vi "Periodic Tasks.vi"(8 "error in":errorcluster) -> ()   [LabVIEW 2015]
doc: "This VI runs in parallel to other tasks. It can contain as many user-defined periodic loops as you need. These can carry out PID or other sorts of timed response."
uses:
  PickupState.ctl
  ShootState.ctl
  TargetState.ctl
  <vilib>/Rock Robotics/WPI/Relay/WPI_RelayValue.ctl
  Robot Global Data.vi
  <vilib>/Rock Robotics/Network Tables/NT Write Numeric Array.vi
  <vilib>/Rock Robotics/WPI/Utilities/WPI_GetSetVariantRefNum.vi
  <vilib>/Rock Robotics/Network Tables/NT Read Numeric Array.vi
  <vilib>/Rock Robotics/WPI/RobotDrive/WPI_RobotDriveArcadeDrive_Standard(NoSaturation).vi
  <vilib>/Rock Robotics/Network Tables/NT Write Boolean Array.vi
  <vilib>/Rock Robotics/Network Tables/NT Read Number.vi
  <vilib>/Rock Robotics/Network Tables/NT Write Number.vi
panel:
  out "aligncount":dbl
  out "Distance (ft)":dbl
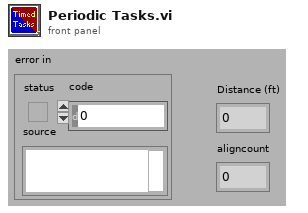
[diagram p1: front panel]
types:
  T1 = typedef "TargetState.ctl" = enum16{"Idle", "CheckVision", "AlignWithTarget", "MoveToTarget", "Wait", "ReAlign", "Stop", "Shoot", "Reset"}
  T2 = typedef "ShootState.ctl" = enum16{"Idle", "Startup", "Fire", "Shutdown", "Startup2"}
  T3 = typedef "PickupState.ctl" = enum16{"Idle", "Intake", "Continue", "Park", "Stop"}
  T4 = typedef "WPI_RelayDevRef.ctl" = cluster{"DevStatus":errorcluster, "Relay Channel":T5, "Relay Direction":T6}
  T5 = typedef "FPGA_DIORelayChannel.ctl" = enum8{"Relay 0", "Relay 1", "Relay 2", "Relay 3", "Invalid"}
  T6 = typedef "WPI_RelayDirection.ctl" = enum16{"Both directions", "Forward only", "Reverse only"}
  T7 = typedef "WPI_EncoderDevRef.ctl" = cluster{"DevStatus":errorcluster, "EncoderIndex":T8, "CounterIndex":T9, "DistancePerCount":dbl, "Decoding Type":T10}
  T8 = typedef "FPGA_EncoderIdx.ctl" = enum8{"Enc 0", "Enc 1", "Enc 2", "Enc 3", "Enc 4", "Enc 5", "Enc 6", "Enc 7", "Invalid"}
  T9 = typedef "FPGA_CounterCtrSystemIndex.ctl" = enum8{"Ctr 0", "Ctr 1", "Ctr 2", "Ctr 3", "Ctr 4", "Ctr 5", "Ctr 6", "Ctr 7", "Invalid"}
  T10 = typedef "WPI_EncoderType.ctl" = enum16{"1x", "2x", "4x"}
  T11 = typedef "WPI_GyroDevRef.ctl" = cluster{"DevStatus":errorcluster, "Analog Channel":T12, "Offset":dbl, "Gain (VoltsPerDegree/Second)":dbl, "Gyro Type":enum16{"Analog", "XRS450"}, "Handle":i32, "SPI Bus":T13, "Device Found":bool, "Sample Rate":dbl, "Calibrate On Open":bool}
  T12 = typedef "FPGA_AIChannel.ctl" = enum8{"AI 0", "AI 1", "AI 2", "AI 3", "AI MXP 0", "AI MXP 1", "AI MXP 2", "AI MXP 3", "Invalid"}
  T13 = typedef "spi_bus.ctl" = enum16{"SPI On-Board, CS0", "SPI On-Board, CS1", "SPI On-Board, CS2", "SPI On-Board, CS3", "SPI MXP", "Invalid"}
  T14 = typedef "WPI_DigitalInputDevRef.ctl" = cluster{"DevStatus":errorcluster, "DIO Channel":T15}
  T15 = typedef "FPGA_DIOChannel.ctl" = enum8{"DIO 0", "DIO 1", "DIO 2", "DIO 3", "DIO 4", "DIO 5", "DIO 6", "DIO 7", "DIO 8", "DIO 9", "DIO MXP 0", "DIO MXP 1", "DIO MXP 2", "DIO MXP 3", "DIO MXP 4", "DIO MXP 5", "DIO MXP 6", "DIO MXP 7", "DIO MXP 8", "DIO MXP 9", "DIO MXP 10", "DIO MXP 11", "DIO MXP 12", "DIO MXP 13", "DIO MXP 14", "DIO MXP 15", "Invalid"}
  T16 = typedef "WPI_RobotDriveDevRef.ctl" = cluster{"DevStatus":errorcluster, "Motors[]":T17[], "Square Inputs":bool, "Max Output":dbl}
  T17 = typedef "WPI_MotorControlDeviceRef.ctl" = cluster{"DeviceStatus":errorcluster, "Type":T18, "PWM":cluster{"PWM Channel":T19, "DeadBand":T20}, "CAN":cluster{"Device Number":u8, "Control Mode":T21, "Semaphore":T22, "Max Vout":dbl, "TalonSRX Control Mode":T23}, "Invert":bool}
  T18 = typedef "WPI_MotorControlType.ctl" = enum16{"PWM", "CAN", "CANTalonSRX"}
  T19 = typedef "FPGA_DIOPWMChannel.ctl" = enum8{"PWM 0", "PWM 1", "PWM 2", "PWM 3", "PWM 4", "PWM 5", "PWM 6", "PWM 7", "PWM 8", "PWM 9", "PWM MXP 0", "PWM MXP 1", "PWM MXP 2", "PWM MXP 3", "PWM MXP 4", "PWM MXP 5", "PWM MXP 6", "PWM MXP 7", "PWM MXP 8", "PWM MXP 9", "Invalid"}
  T20 = typedef "WPI_PWMDeadband.ctl" = cluster{"Name":string, "maxPositivePwm":i32, "minPositivePwm":i32, "centerPwm":i32, "maxNegativePwm":i32, "minNegativePwm":i32, "angularRange":u16}
  T21 = typedef "WPI_CANJaguar_ControlMode.ctl" = enum8{"Percent VBus", "Current", "Speed", "Position", "Voltage"}
  T22 = typedef "Semaphore RefNum" = refnum<k1>
  T23 = typedef "WPI_CANTalonSRX_APIControlMode.ctl" = enum8{"Percent VBus", "Speed", "Position", "Slave", "Unchanged / Invalid", "Voltage Compensation", "Current", "Motion Profile"}
  T24 = typedef "WPI_RelayValue.ctl" = enum16{"Off", "On", "Forward", "Reverse"}
  T25 = cluster{"Distance (ft)":dbl, "Center":cluster{dbl, dbl}, "Normalized Rect":cluster{"Numeric":dbl, "Numeric 2":dbl, "Numeric 3":dbl, "Numeric 5":dbl}}[]
  T26 = cluster{"Distance (ft)":dbl, "Center":cluster{dbl, dbl}, "Normalized Rect":cluster{"Numeric":dbl, "Numeric 2":dbl, "Numeric 3":dbl, "Numeric 5":dbl}}
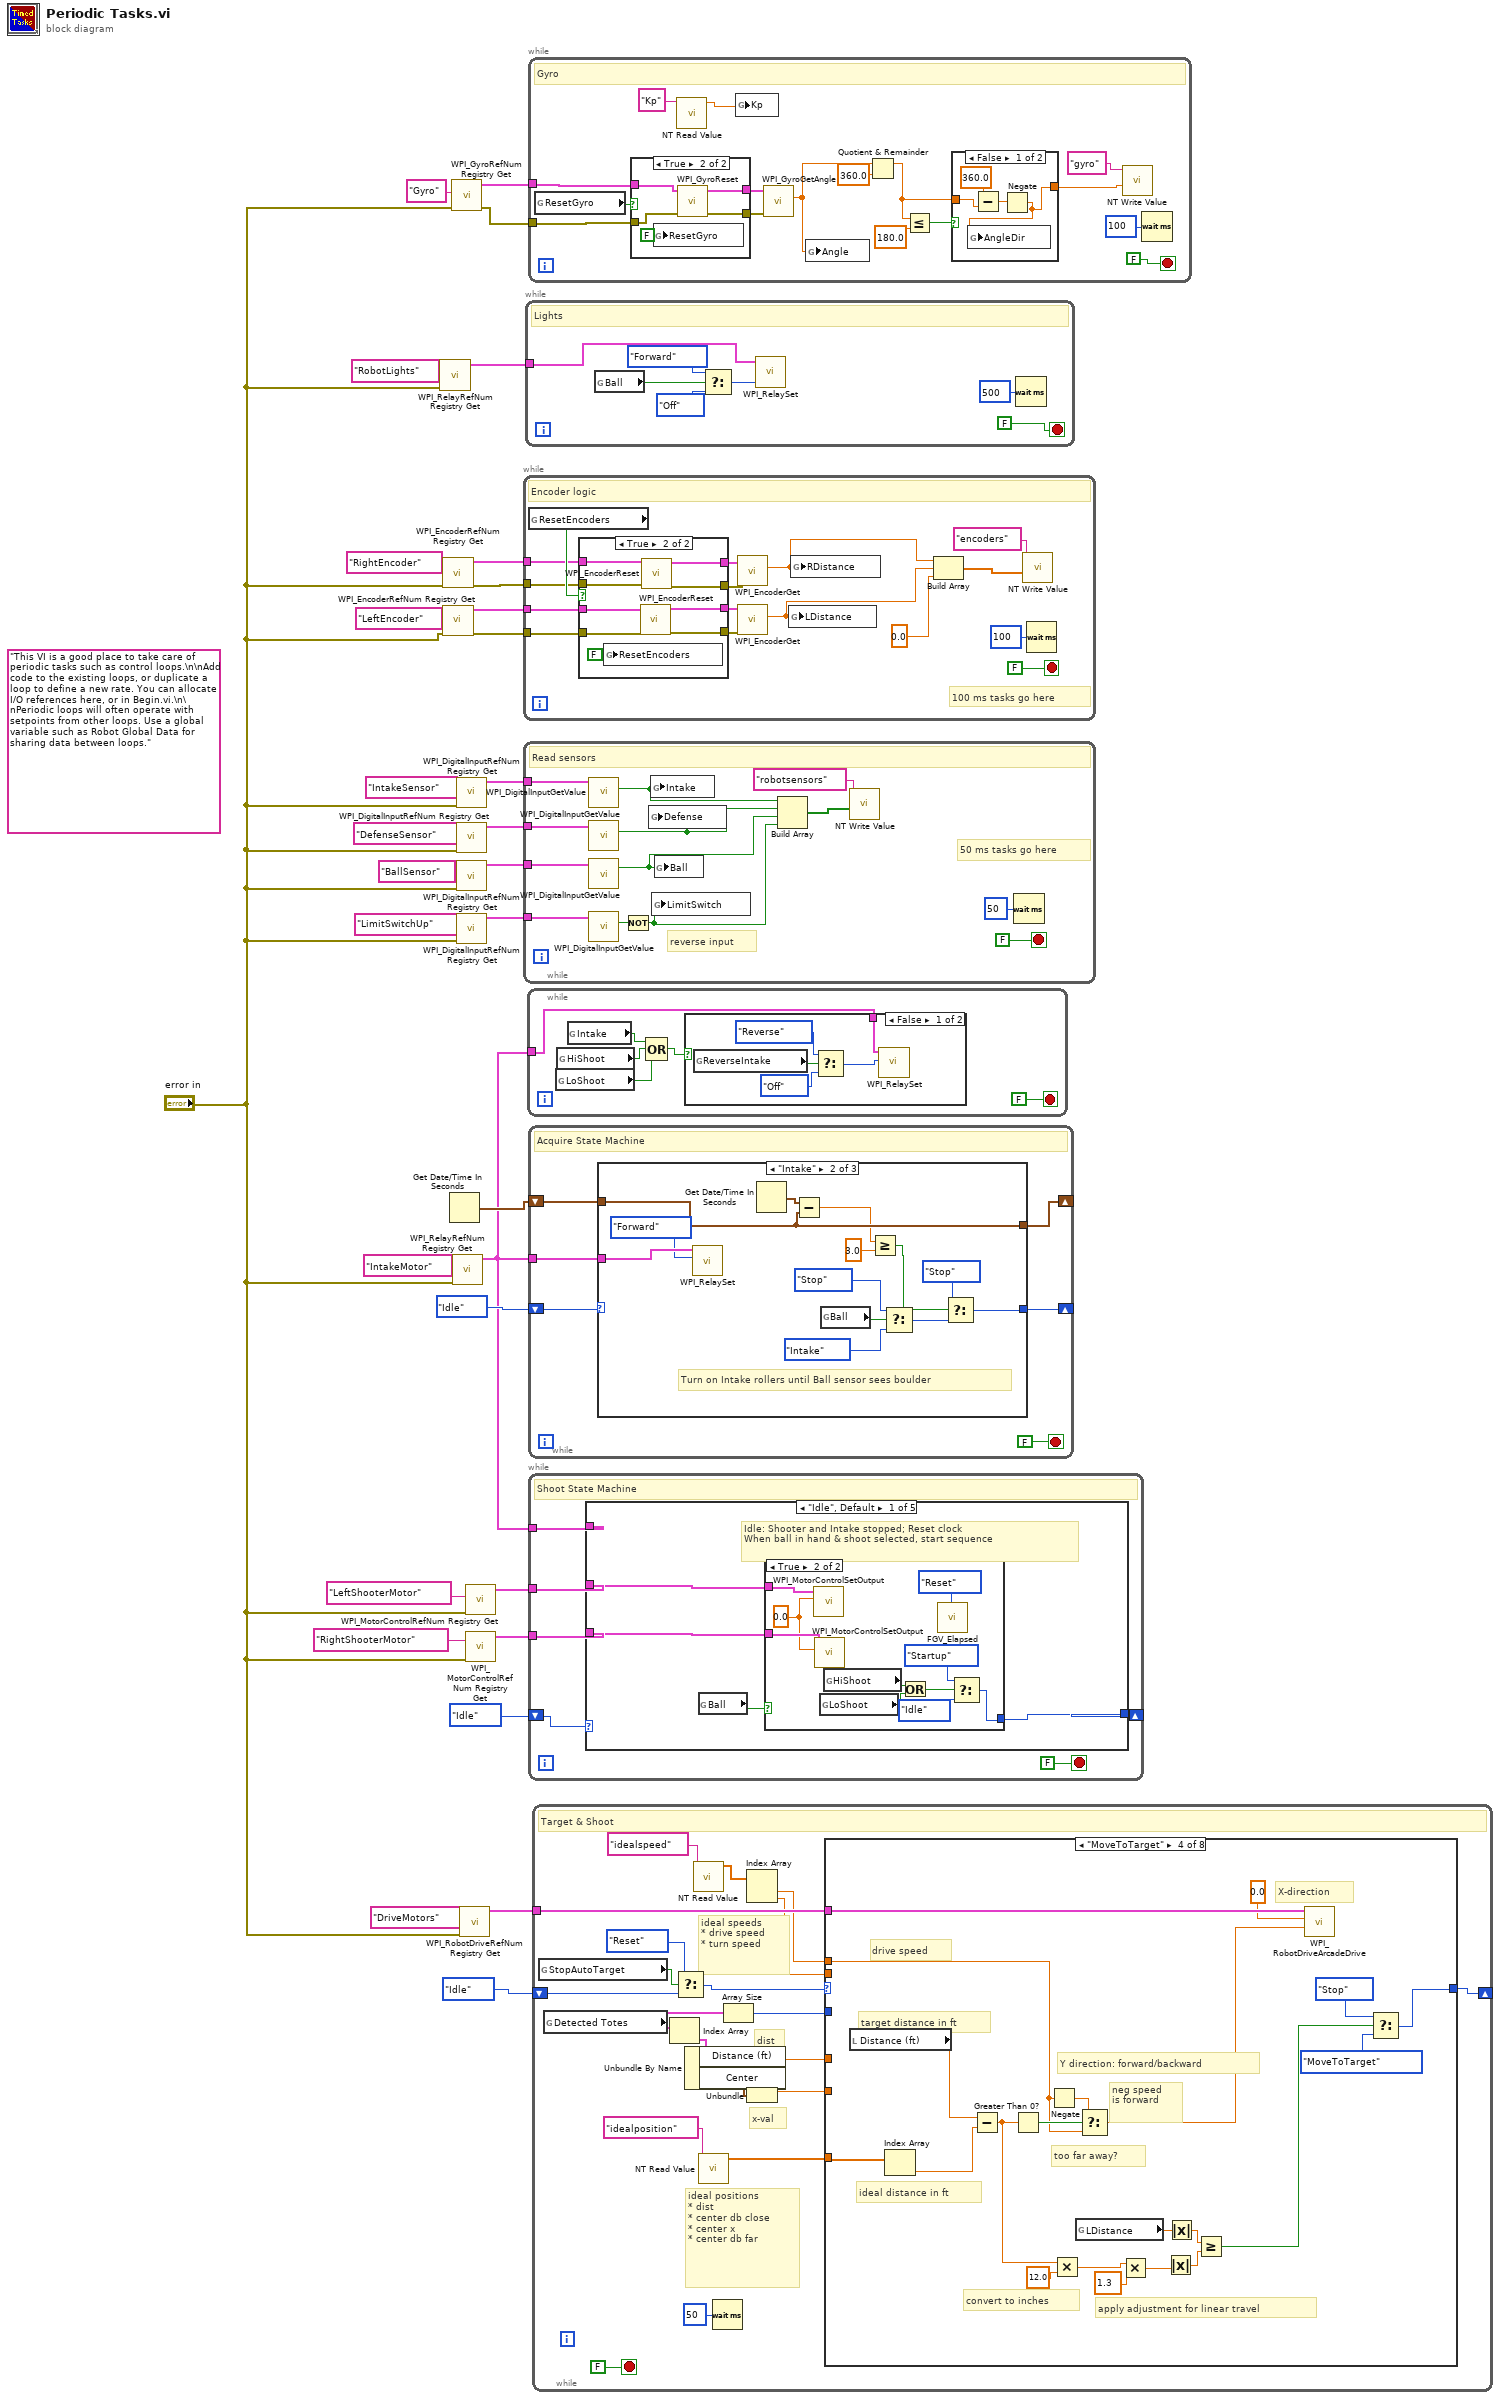
[diagram p0: block diagram]
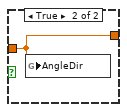
[diagram p2: hidden frame]
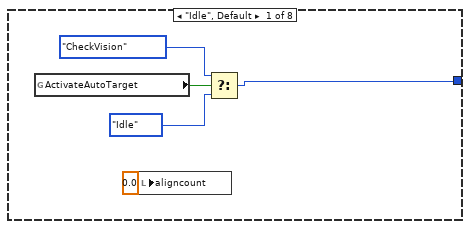
[diagram p5: hidden frame]
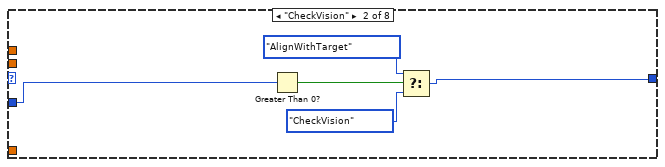
[diagram p6: hidden frame]
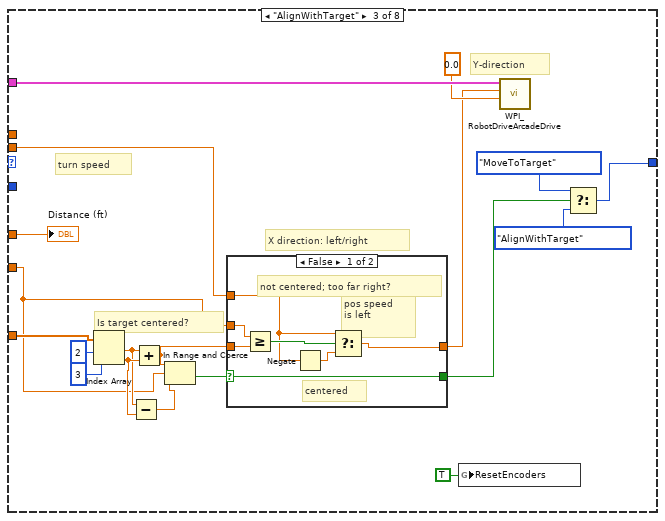
[diagram p7: hidden frame]
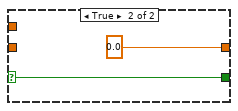
[diagram p8: hidden frame]
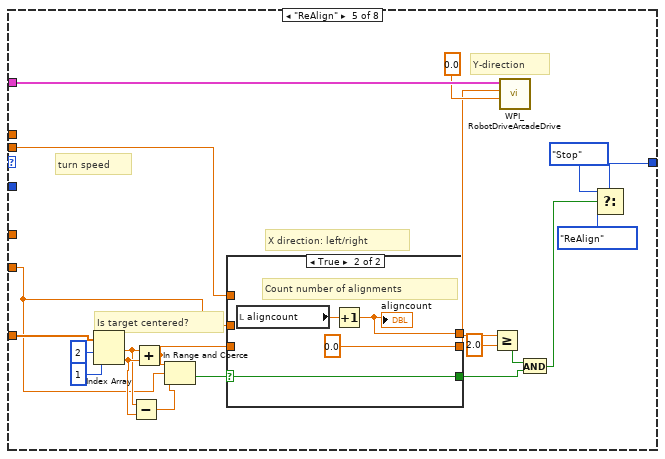
[diagram p9: hidden frame]
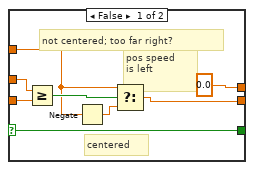
[diagram p10: hidden frame]
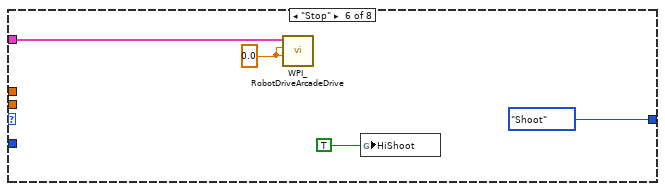
[diagram p11: hidden frame]
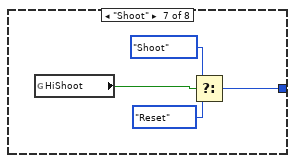
[diagram p12: hidden frame]
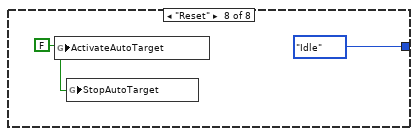
[diagram p13: hidden frame]
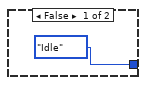
[diagram p14: hidden frame]
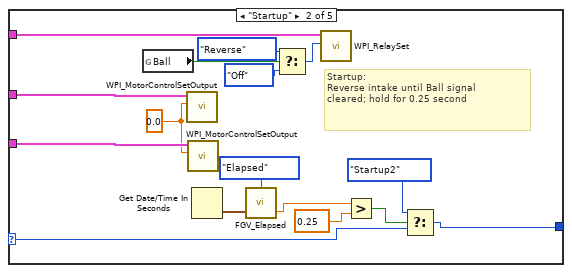
[diagram p15: hidden frame]
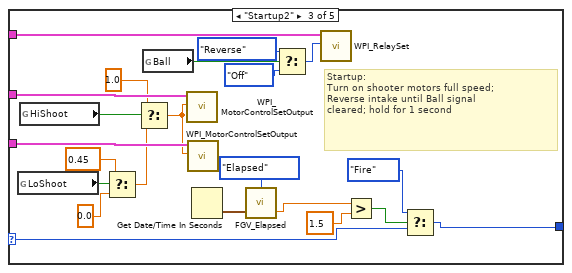
[diagram p16: hidden frame]
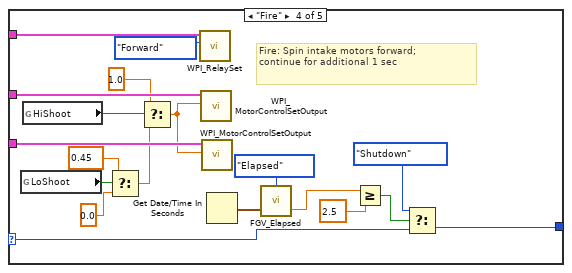
[diagram p17: hidden frame]
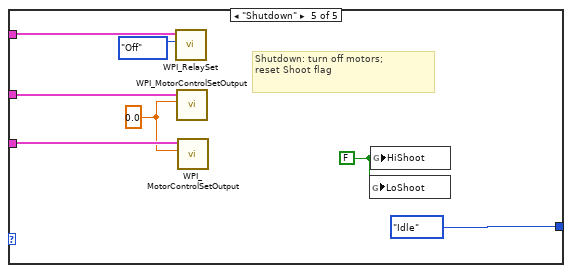
[diagram p18: hidden frame]
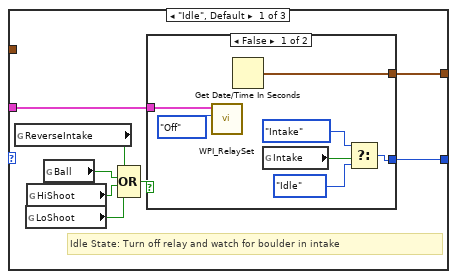
[diagram p19: hidden frame]
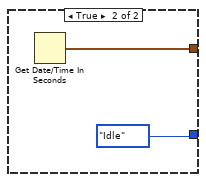
[diagram p20: hidden frame]
diagram:
  (unwired) "This VI is a good place to take care of periodic tasks such as control loops.\n\nAdd code to the existing loops, or duplicate a loop to define a new rate. You can allocate I/O references here, or in Begin.vi.\n\nPeriodic loops will often operate with setpoints from other loops. Use a global variable such as Robot Global Data for sharing data between loops."
  n1 = call <vilib>:"WPI_RelayRefNum Registry Get.vi"("error in (no error)"="error in", "refnum name"="RobotLights") -> ("RelayDevRef"=w14:T4)  [unwired: 8 in, 1 out]
  n2 = call <vilib>:"WPI_EncoderRefNum Registry Get.vi"("error in (no error)"="error in", "refnum name"="RightEncoder") -> ("error out"=w30:errorcluster, "EncoderDevRef"=w31:T7)  [unwired: 8 in]
  n3 = call <vilib>:"WPI_EncoderRefNum Registry Get.vi"("error in (no error)"="error in", "refnum name"="LeftEncoder") -> ("error out"=w29:errorcluster, "EncoderDevRef"=w32:T7)  [unwired: 8 in]
  n4 = Get Date/Time In Seconds() -> (seconds since 1Jan1904=w6:timestamp)
  n5 = call <vilib>:"WPI_GyroRefNum Registry Get.vi"("error in (no error)"="error in", "refnum name"="Gyro") -> ("error out"=w2:errorcluster, "GyroDevRef"=w3:T11)  [unwired: 8 in]
  n6 = call <vilib>:"WPI_RelayRefNum Registry Get.vi"("error in (no error)"="error in", "refnum name"="IntakeMotor") -> ("RelayDevRef"=w5:T4)  [unwired: 8 in, 1 out]
  n7 = call <vilib>:"WPI_DigitalInputRefNum Registry Get.vi"("error in (no error)"="error in", "refnum name"="IntakeSensor") -> ("DigitalInputDevRef"=w24:T14)  [unwired: 8 in, 1 out]
  n8 = call <vilib>:"WPI_DigitalInputRefNum Registry Get.vi"("error in (no error)"="error in", "refnum name"="DefenseSensor") -> ("DigitalInputDevRef"=w10:T14)  [unwired: 8 in, 1 out]
  n9 = call <vilib>:"WPI_DigitalInputRefNum Registry Get.vi"("error in (no error)"="error in", "refnum name"="BallSensor") -> ("DigitalInputDevRef"=w16:T14)  [unwired: 8 in, 1 out]
  n10 = call <vilib>:"WPI_DigitalInputRefNum Registry Get.vi"("error in (no error)"="error in", "refnum name"="LimitSwitchUp") -> ("DigitalInputDevRef"=w7:T14)  [unwired: 8 in, 1 out]
  n11 = call <vilib>:"WPI_RobotDriveRefNum Registry Get.vi"("error in (no error)"="error in", "refnum name"="DriveMotors") -> ("RobotDriveDevRef"=w11:T16)  [unwired: 8 in, 1 out]
  n12 = call <vilib>:"WPI_MotorControlRefNum Registry Get.vi"("error in (no error)"="error in", "refnum name"="LeftShooterMotor") -> ("MotorControlDevRef"=w19:T17)  [unwired: 8 in, 1 out]
  n13 = call <vilib>:"WPI_MotorControlRefNum Registry Get.vi"("error in (no error)"="error in", "refnum name"="RightShooterMotor") -> ("MotorControlDevRef"=w18:T17)  [unwired: 8 in, 1 out]
  n14 = while {
    tunnel: w32 -> [w37]
    tunnel: w31 -> [w41]
    tunnel: w30 -> [w39]
    tunnel: w29 -> [w36]
    stop <- FALSE stop-if-true
    # "100 ms tasks go here"
    # "Encoder logic"
    n15 = global read "Robot Global Data.vi" "ResetEncoders"() -> (w42:bool)
    n16 = case shown="True" w42 {
      tunnel: w41 -> [w52 w61]
      tunnel: [w52 w60] -> w40
      tunnel: w39 -> [w51 w59]
      tunnel: [w51 w58] -> w38
      tunnel: w37 -> [w50 w57]
      tunnel: w36 -> [w49 w56]
      tunnel: [w50 w55] -> w35
      tunnel: [w49 w54] -> w34
      frame False {
      }
      frame True {
        n17 = global write "Robot Global Data.vi" "ResetEncoders"(FALSE) -> ()
        n18 = call <vilib>:"WPI_EncoderReset.vi"("error in (no error)"=w56, "EncoderDevRef"=w57) -> ("error out"=w54:errorcluster, "EncoderDevRef"=w55:T7)  [unwired: 8 in]
        n19 = call <vilib>:"WPI_EncoderReset.vi"("error in (no error)"=w59, "EncoderDevRef"=w61) -> ("error out"=w58:errorcluster, "EncoderDevRef"=w60:T7)  [unwired: 8 in]
      }
    }
    n20 = call <vilib>:"WPI_EncoderGet.vi"("error in (no error)"=w38, "EncoderDevRef"=w40) -> ("Distance"=w44:dbl)  [unwired: 4 in, 5 out]
    n21 = call <vilib>:"WPI_EncoderGet.vi"("error in (no error)"=w34, "EncoderDevRef"=w35) -> ("Distance"=w43:dbl)  [unwired: 4 in, 5 out]
    n22 = global write "Robot Global Data.vi" "LDistance"(w43) -> ()
    n23 = global write "Robot Global Data.vi" "RDistance"(w44) -> ()
    n24 = Build Array(w44, w43, 0.0) -> (w46:dbl[])
    n25 = call-poly <vilib>:"NT Write Value.vi"("Numeric Array"=w46, "Name"="encoders") -> ()  [unwired: 9 in, 1 out]
    n26 = Wait (ms)(milliseconds to wait=u32 100) -> ()  [unwired: 1 out]
  }
  n27 = while {
    tunnel: w24 -> [w72]
    tunnel: w16 -> [w68]
    tunnel: w10 -> [w66]
    tunnel: w7 -> [w65]
    stop <- FALSE stop-if-true
    # "reverse input"
    # "50 ms tasks go here"
    # "Read sensors"
    n28 = call <vilib>:"WPI_DigitalInputGetValue.vi"("DigitalInputDevRef"=w72) -> ("Value"=w71:bool)  [unwired: 8 in, 2 out]
    n29 = call <vilib>:"WPI_DigitalInputGetValue.vi"("DigitalInputDevRef"=w66) -> ("Value"=w63:bool)  [unwired: 8 in, 2 out]
    n30 = call <vilib>:"WPI_DigitalInputGetValue.vi"("DigitalInputDevRef"=w68) -> ("Value"=w67:bool)  [unwired: 8 in, 2 out]
    n31 = call <vilib>:"WPI_DigitalInputGetValue.vi"("DigitalInputDevRef"=w65) -> ("Value"=w64:bool)  [unwired: 8 in, 2 out]
    n32 = Not(x=w64) -> (.not. x?=w62:bool)
    n33 = global write "Robot Global Data.vi" "Defense"(w63) -> ()
    n34 = global write "Robot Global Data.vi" "Intake"(w71) -> ()
    n35 = global write "Robot Global Data.vi" "LimitSwitch"(w62) -> ()
    n36 = global write "Robot Global Data.vi" "Ball"(w67) -> ()
    n37 = Build Array(w71, w63, w67, w62) -> (w70:bool[])
    n38 = call-poly <vilib>:"NT Write Value.vi"("Boolean Array"=w70, "Name"="robotsensors") -> ()  [unwired: 9 in, 1 out]
    n39 = Wait (ms)(milliseconds to wait=u32 50) -> ()  [unwired: 1 out]
  }
  n40 = while {
    tunnel: w14 -> [w78]
    stop <- FALSE stop-if-true
    # "Lights"
    n41 = global read "Robot Global Data.vi" "Ball"() -> (w77:bool)
    n42 = Select(t=WPI_RelayValue."Forward" ("RelayValue"), s=w77, f=WPI_RelayValue."Off" ("RelayValue")) -> (s? t:f=w81:T24)
    n43 = call <vilib>:"WPI_RelaySet.vi"("RelayValue"=w81, "RelayDevRef"=w78) -> ()  [unwired: 8 in, 2 out]
    n44 = Wait (ms)(milliseconds to wait=u32 500) -> ()  [unwired: 1 out]
  }
  n45 = while {
    tunnel: w5 -> [w86]
    stop <- FALSE stop-if-true
    n46 = global read "Robot Global Data.vi" "LoShoot"() -> (w85:bool)
    n47 = global read "Robot Global Data.vi" "HiShoot"() -> (w84:bool)
    n48 = global read "Robot Global Data.vi" "Intake"() -> (w82:bool)
    n49 = Compound Arithmetic op=OR(w82, w84, w85) -> (w83:bool)
    n50 = case shown="False" w83 {
      tunnel: w86 -> [w92 _]
      frame False {
        n51 = global read "Robot Global Data.vi" "ReverseIntake"() -> (w88:bool)
        n52 = Select(t=WPI_RelayValue."Reverse" ("RelayValue"), s=w88, f=WPI_RelayValue."Off" ("RelayValue")) -> (s? t:f=w89:T24)
        n53 = call <vilib>:"WPI_RelaySet.vi"("RelayValue"=w89, "RelayDevRef"=w92) -> ()  [unwired: 8 in, 2 out]
      }
      frame True {
      }
    }
  }
  n54 = while {
    tunnel: w3 -> [w108]
    tunnel: w2 -> [w106]
    stop <- FALSE stop-if-true
    # "Gyro"
    n55 = global read "Robot Global Data.vi" "ResetGyro"() -> (w104:bool)
    n56 = case shown="True" w104 {
      tunnel: w108 -> [w114 w120]
      tunnel: [w114 w119] -> w107
      tunnel: w106 -> [w115 w118]
      tunnel: [w115 w117] -> w105
      frame False {
      }
      frame True {
        n57 = global write "Robot Global Data.vi" "ResetGyro"(FALSE) -> ()
        n58 = call <vilib>:"WPI_GyroReset.vi"("error in"=w118, "GyroDevRef"=w120) -> ("error out"=w117:errorcluster, "GyroDevRef"=w119:T11)  [unwired: 8 in]
      }
    }
    n59 = call-poly <vilib>:"NT Read Value.vi"("Name"="Kp") -> ("Numeric"=w93:dbl)  [unwired: 9 in, 1 out]
    n60 = global write "Robot Global Data.vi" "Kp"(w93) -> ()
    n61 = call <vilib>:"WPI_GyroGetAngle.vi"("error in"=w105, "GyroDevRef"=w107) -> ("Angle"=w101:dbl)  [unwired: 5 in, 4 out]
    n62 = global write "Robot Global Data.vi" "Angle"(w101) -> ()
    n63 = Quotient & Remainder(x=w101, y=360.0) -> (x-y*floor(x/y)=w96:dbl)  [unwired: 1 out]
    n64 = Less Or Equal?(x=w96, y=180.0) -> (x <= y?=w98:bool)
    n65 = case shown="False" w98 {
      tunnel: w96 -> [w111 w113]
      tunnel: [w109 w113] -> w95
      frame False {
        n66 = Subtract(x=360.0 ("y"), y=w111) -> (x-y=w110:dbl)
        n67 = Negate(x=w110) -> (-x=w109:dbl)
        n68 = global write "Robot Global Data.vi" "AngleDir"(w109) -> ()
      }
      frame True {
        n69 = global write "Robot Global Data.vi" "AngleDir"(w113) -> ()
      }
    }
    n70 = call-poly <vilib>:"NT Write Value.vi"("Numeric"=w95, "Name"="gyro") -> ()  [unwired: 9 in, 1 out]
    n71 = Wait (ms)(milliseconds to wait=u32 100) -> ()  [unwired: 1 out]
  }
  n72 = while {
    shift-right: [w123] -> _
    shift-left: PickupState."Idle" ("PickupState") -> [w125]
    tunnel: w5 -> [w124]
    shift-right: [w122] -> _
    shift-left: w6 -> [w121]
    stop <- FALSE stop-if-true
    # "Acquire State Machine"
    n73 = case shown="\"Intake\"" w125 {
      tunnel: w124 -> [w133 w156 w160]
      tunnel: [w134 w151 PickupState."Idle" ("PickupState")] -> w123
      tunnel: [w132 w147 w157] -> w122
      tunnel: w121 -> [_ w147 w157]
      frame "Idle", Default {
        # "Idle State: Turn off relay and watch for boulder in intake"
        n74 = global read "Robot Global Data.vi" "ReverseIntake"() -> (w127:bool)
        n75 = global read "Robot Global Data.vi" "LoShoot"() -> (w128:bool)
        n76 = global read "Robot Global Data.vi" "HiShoot"() -> (w129:bool)
        n77 = global read "Robot Global Data.vi" "Ball"() -> (w130:bool)
        n78 = Compound Arithmetic op=OR(w127, w130, w129, w128) -> (w131:bool)
        n79 = case shown="False" w131 {
          tunnel: [w140 PickupState."Idle" ("PickupState")] -> w134
          tunnel: w133 -> [w138 _]
          tunnel: [w135 w142] -> w132
          frame False {
            n80 = call <vilib>:"WPI_RelaySet.vi"("RelayValue"=WPI_RelayValue."Off", "RelayDevRef"=w138) -> ()  [unwired: 8 in, 2 out]
            n81 = Get Date/Time In Seconds() -> (seconds since 1Jan1904=w135:timestamp)
            n82 = global read "Robot Global Data.vi" "Intake"() -> (w141:bool)
            n83 = Select(t=PickupState."Intake" ("PickupState"), s=w141, f=PickupState."Idle" ("PickupState")) -> (s? t:f=w140:T3)
          }
          frame True {
            n84 = Get Date/Time In Seconds() -> (seconds since 1Jan1904=w142:timestamp)
          }
        }
      }
      frame "Intake" {
        # "Turn on Intake rollers until Ball sensor sees boulder"
        n85 = call <vilib>:"WPI_RelaySet.vi"("RelayValue"=WPI_RelayValue."Forward", "RelayDevRef"=w156) -> ()  [unwired: 8 in, 2 out]
        n86 = Get Date/Time In Seconds() -> (seconds since 1Jan1904=w148:timestamp)
        n87 = Subtract(x=w148, y=w147) -> (x-y=w146:dbl)
        n88 = global read "Robot Global Data.vi" "Ball"() -> (w154:bool)
        n89 = Greater Or Equal?(x=w146, y=3.0) -> (x >= y?=w144:bool)
        n90 = Select(t=PickupState."Stop" ("PickupState"), s=w154, f=PickupState."Intake" ("PickupState")) -> (s? t:f=w150:T3)
        n91 = Select(t=PickupState."Stop" ("PickupState"), s=w144, f=w150) -> (s? t:f=w151:T3)
      }
      frame "Stop" {
        # "Stop the motor"
        n92 = call <vilib>:"WPI_RelaySet.vi"("RelayValue"=WPI_RelayValue."Off", "RelayDevRef"=w160) -> ()  [unwired: 8 in, 2 out]
      }
    }
  }
  n93 = while {
    shift-right: [w162] -> _
    shift-left: ShootState."Idle" ("ShootState") -> [w166]
    tunnel: w5 -> [w161]
    tunnel: w19 -> [w164]
    tunnel: w18 -> [w163]
    stop <- FALSE stop-if-true
    # "Shoot State Machine"
    n94 = case shown="\"Idle\", Default" w166 {
      selector: w166 -> [_ w193 w215 w231 _]
      tunnel: w164 -> [w170 w197 w219 w238 w245]
      tunnel: w163 -> [w169 w196 w218 w237 w244]
      tunnel: [w168 w192 w214 w233 ShootState."Idle" ("ShootState")] -> w162
      tunnel: w161 -> [_ w187 w209 w236 w243]
      frame "Idle", Default {
        # "Idle: Shooter and Intake stopped; Reset clock\nWhen ball in hand & shoot selected, start sequence"
        n95 = global read "Robot Global Data.vi" "Ball"() -> (w167:bool)
        n96 = case shown="True" w167 {
          tunnel: w170 -> [_ w181]
          tunnel: w169 -> [_ w180]
          tunnel: [ShootState."Idle" ("ShootState") w178] -> w168
          frame False {
          }
          frame True {
            w179 = 0.0 ("Output")
            n97 = call <vilib>:"WPI_MotorControlSetOutput.vi"("Output"=w179, "MotorControlDevRef"=w181) -> ()  [unwired: 7 in, 3 out]
            n98 = call <vilib>:"WPI_MotorControlSetOutput.vi"("Output"=w179, "MotorControlDevRef"=w180) -> ()  [unwired: 7 in, 3 out]
            n99 = global read "Robot Global Data.vi" "LoShoot"() -> (w173:bool)
            n100 = global read "Robot Global Data.vi" "HiShoot"() -> (w174:bool)
            n101 = Or(x=w174, y=w173) -> (x .or. y?=w172:bool)
            n102 = call "FGV_Elapsed.vi"("Function"=enum16{"Elapsed", "Reset"}."Reset") -> ()  [unwired: 1 in, 1 out]
            n103 = Select(t=ShootState."Startup" ("ShootState"), s=w172, f=ShootState."Idle" ("ShootState")) -> (s? t:f=w178:T2)
          }
        }
      }
      frame "Startup" {
        w182 = 0.0 ("f")
        # "Startup:\nReverse intake until Ball signal\ncleared; hold for 0.25 second"
        n104 = global read "Robot Global Data.vi" "Ball"() -> (w186:bool)
        n105 = call <vilib>:"WPI_MotorControlSetOutput.vi"("Output"=w182, "MotorControlDevRef"=w197) -> ()  [unwired: 7 in, 3 out]
        n106 = call <vilib>:"WPI_MotorControlSetOutput.vi"("Output"=w182, "MotorControlDevRef"=w196) -> ()  [unwired: 7 in, 3 out]
        n107 = Get Date/Time In Seconds() -> (seconds since 1Jan1904=w190:timestamp)
        n108 = call "FGV_Elapsed.vi"("Function"=enum16{"Elapsed", "Reset"}."Elapsed", "DateTime"=w190) -> ("Elapsed"=w189:dbl)
        n109 = Select(t=WPI_RelayValue."Reverse" ("RelayValue"), s=w186, f=WPI_RelayValue."Off" ("RelayValue")) -> (s? t:f=w183:T24)
        n110 = call <vilib>:"WPI_RelaySet.vi"("RelayValue"=w183, "RelayDevRef"=w187) -> ()  [unwired: 8 in, 2 out]
        n111 = Greater?(x=w189, y=0.25) -> (0:w194:bool)
        n112 = Select(t=ShootState."Startup2" ("ShootState"), s=w194, f=w193) -> (s? t:f=w192:T2)
      }
      frame "Startup2" {
        # "Startup:\nTurn on shooter motors full speed;\nReverse intake until Ball signal\ncleared; hold for 1 second"
        n113 = global read "Robot Global Data.vi" "LoShoot"() -> (w202:bool)
        n114 = global read "Robot Global Data.vi" "HiShoot"() -> (w204:bool)
        n115 = Select(t=0.45, s=w202, f=0.0) -> (s? t:f=w200:dbl)
        n116 = Select(t=1.0, s=w204, f=w200) -> (s? t:f=w198:dbl)
        n117 = global read "Robot Global Data.vi" "Ball"() -> (w208:bool)
        n118 = call <vilib>:"WPI_MotorControlSetOutput.vi"("Output"=w198, "MotorControlDevRef"=w219) -> ()  [unwired: 7 in, 3 out]
        n119 = call <vilib>:"WPI_MotorControlSetOutput.vi"("Output"=w198, "MotorControlDevRef"=w218) -> ()  [unwired: 7 in, 3 out]
        n120 = Get Date/Time In Seconds() -> (seconds since 1Jan1904=w212:timestamp)
        n121 = call "FGV_Elapsed.vi"("Function"=enum16{"Elapsed", "Reset"}."Elapsed", "DateTime"=w212) -> ("Elapsed"=w211:dbl)
        n122 = Select(t=WPI_RelayValue."Reverse" ("RelayValue"), s=w208, f=WPI_RelayValue."Off" ("RelayValue")) -> (s? t:f=w205:T24)
        n123 = call <vilib>:"WPI_RelaySet.vi"("RelayValue"=w205, "RelayDevRef"=w209) -> ()  [unwired: 8 in, 2 out]
        n124 = Greater?(x=w211, y=1.5) -> (0:w216:bool)
        n125 = Select(t=ShootState."Fire" ("ShootState"), s=w216, f=w215) -> (s? t:f=w214:T2)
      }
      frame "Fire" {
        # "Fire: Spin intake motors forward;\ncontinue for additional 1 sec"
        n126 = global read "Robot Global Data.vi" "LoShoot"() -> (w224:bool)
        n127 = global read "Robot Global Data.vi" "HiShoot"() -> (w226:bool)
        n128 = Select(t=0.45, s=w224, f=0.0) -> (s? t:f=w222:dbl)
        n129 = Select(t=1.0, s=w226, f=w222) -> (s? t:f=w221:dbl)
        n130 = call <vilib>:"WPI_RelaySet.vi"("RelayValue"=WPI_RelayValue."Forward", "RelayDevRef"=w236) -> ()  [unwired: 8 in, 2 out]
        n131 = call <vilib>:"WPI_MotorControlSetOutput.vi"("Output"=w221, "MotorControlDevRef"=w238) -> ()  [unwired: 7 in, 3 out]
        n132 = call <vilib>:"WPI_MotorControlSetOutput.vi"("Output"=w221, "MotorControlDevRef"=w237) -> ()  [unwired: 7 in, 3 out]
        n133 = Get Date/Time In Seconds() -> (seconds since 1Jan1904=w229:timestamp)
        n134 = call "FGV_Elapsed.vi"("Function"=enum16{"Elapsed", "Reset"}."Elapsed", "DateTime"=w229) -> ("Elapsed"=w227:dbl)
        n135 = Greater Or Equal?(x=w227, y=2.5) -> (x >= y?=w232:bool)
        n136 = Select(t=ShootState."Shutdown" ("ShootState"), s=w232, f=w231) -> (s? t:f=w233:T2)
      }
      frame "Shutdown" {
        w239 = FALSE
        w242 = 0.0 ("Output")
        # "Shutdown: turn off motors;\nreset Shoot flag"
        n137 = call <vilib>:"WPI_RelaySet.vi"("RelayValue"=WPI_RelayValue."Off", "RelayDevRef"=w243) -> ()  [unwired: 8 in, 2 out]
        n138 = call <vilib>:"WPI_MotorControlSetOutput.vi"("Output"=w242, "MotorControlDevRef"=w245) -> ()  [unwired: 7 in, 3 out]
        n139 = call <vilib>:"WPI_MotorControlSetOutput.vi"("Output"=w242, "MotorControlDevRef"=w244) -> ()  [unwired: 7 in, 3 out]
        n140 = global write "Robot Global Data.vi" "LoShoot"(w239) -> ()
        n141 = global write "Robot Global Data.vi" "HiShoot"(w239) -> ()
      }
    }
  }
  n142 = while {
    shift-right: [w251] -> _
    shift-left: TargetState."Idle" ("TargetState") -> [w249]
    tunnel: w11 -> [w258]
    stop <- FALSE stop-if-true
    # "ideal speeds\n* drive speed\n* turn speed"
    # "ideal positions\n* dist\n* center db close\n* center x\n* center db far"
    # "x-val"
    # "dist"
    # "Target & Shoot"
    n143 = global read "Robot Global Data.vi" "StopAutoTarget"() -> (w250:bool)
    n144 = global read "Robot Global Data.vi" "Detected Totes"() -> (w261:T25)
    n145 = Index Array(array=w261) -> (element=w263:T26)  [unwired: 1 in]
    n146 = Select(t=TargetState."Reset" ("TargetState"), s=w250, f=w249) -> (s? t:f=w248:T1)
    n147 = Unbundle By Name(w263) -> ("Distance (ft)"=w253:dbl, "Center"=w264:cluster{dbl, dbl})
    n148 = call-poly <vilib>:"NT Read Value.vi"("Name"="idealspeed") -> ("Numeric Array"=w259:dbl[])  [unwired: 9 in, 1 out]
    n149 = call-poly <vilib>:"NT Read Value.vi"("Name"="idealposition") -> ("Numeric Array"=w256:dbl[])  [unwired: 9 in, 1 out]
    n150 = Wait (ms)(milliseconds to wait=u32 50) -> ()  [unwired: 1 out]
    n151 = Array Size(array=w261) -> (size(s)=w252:i32)
    n152 = Index Array(array=w259) -> (element #1=w257:dbl, element #2=w255:dbl)  [unwired: 2 in]
    n153 = Unbundle(w264) -> (w254:dbl)  [unwired: 1 out]
    n154 = case shown="\"MoveToTarget\"" w248 {
      tunnel: w258 -> [_ _ w294 w324 w345 w361 _ _]
      tunnel: w257 -> [_ _ _ w316 _ _ _ _]
      tunnel: w256 -> [_ _ w286 w319 w337 _ _ _]
      tunnel: w255 -> [_ _ w284 _ w335 _ _ _]
      tunnel: w254 -> [_ _ w285 _ w336 _ _ _]
      tunnel: w253 -> [_ _ w276 _ _ _ _ _]
      tunnel: w252 -> [_ w275 _ _ _ _ _ _]
      tunnel: [w267 w271 w279 w322 w331 TargetState."Shoot" ("TargetState") w362 TargetState."Idle" ("TargetState")] -> w251
      frame "Idle", Default {
        n155 = global read "Robot Global Data.vi" "ActivateAutoTarget"() -> (w270:bool)
        n156 = local write "aligncount"(0.0 ("aligncount")) -> ()
        n157 = Select(t=TargetState."CheckVision" ("TargetState"), s=w270, f=TargetState."Idle" ("TargetState")) -> (s? t:f=w267:T1)
      }
      frame "CheckVision" {
        n158 = Greater Than 0?(x=w275) -> (x > 0?=w274:bool)
        n159 = Select(t=TargetState."AlignWithTarget" ("TargetState"), s=w274, f=TargetState."CheckVision" ("TargetState")) -> (s? t:f=w271:T1)
      }
      frame "AlignWithTarget" {
        # "Y-direction"
        # "turn speed"
        # "X direction: left/right"
        # "Is target centered?"
        n160 = Index Array(array=w286, index #1=2 ("index"), index #2=3 ("index")) -> (element #1=w291:dbl, element #2=w292:dbl)
        n161 = Subtract(x=w291, y=w292) -> (x-y=w290:dbl)
        n162 = Add(x=w291, y=w292) -> (x+y=w293:dbl)
        n163 = In Range and Coerce(upper limit=w293, x=w285, lower limit=w290) -> (In Range?=w287:bool)  [unwired: 1 out]
        n164 = case shown="False" w287 {
          selector: w287 -> [w301 w303]
          tunnel: [w301 w303] -> w281
          tunnel: [w299 0.0] -> w282
          tunnel: w285 -> [w298 _]
          tunnel: w293 -> [w297 _]
          tunnel: w284 -> [w295 _]
          frame False {
            # "centered"
            # "pos speed\nis left"
            # "not centered; too far right?"
            n165 = Greater Or Equal?(x=w298, y=w297) -> (x >= y?=w300:bool)
            n166 = Negate(x=w295) -> (-x=w296:dbl)
            n167 = Select(t=w295, s=w300, f=w296) -> (s? t:f=w299:dbl)
          }
          frame True {
          }
        }
        n168 = global write "Robot Global Data.vi" "ResetEncoders"(TRUE) -> ()
        n169 = call-poly <vilib>:"WPI_RobotDriveArcadeDrive.vi"("Y axis value"=0.0, "X axis value"=w282, "RobotDriveDevRef"=w294) -> ()  [unwired: 6 in, 3 out]
        n170 = Select(t=TargetState."MoveToTarget" ("TargetState"), s=w281, f=TargetState."AlignWithTarget" ("TargetState")) -> (s? t:f=w279:T1)
        "Distance (ft)" <- w276
      }
      frame "MoveToTarget" {
        # "apply adjustment for linear travel"
        # "target distance in ft"
        # "ideal distance in ft"
        # "convert to inches"
        # "too far away?"
        # "neg speed\nis forward"
        # "X-direction"
        # "drive speed"
        # "Y direction: forward/backward"
        n171 = local read "Distance (ft)"() -> (w310:dbl)
        n172 = Index Array(array=w319) -> (element=w309:dbl)  [unwired: 1 in]
        n173 = Subtract(x=w310, y=w309) -> (x-y=w308:dbl)
        n174 = Greater Than 0?(x=w308) -> (x > 0?=w318:bool)
        n175 = Negate(x=w316) -> (-x=w317:dbl)
        n176 = Multiply(x=w308, y=12.0) -> (x*y=w305:dbl)
        n177 = global read "Robot Global Data.vi" "LDistance"() -> (w314:dbl)
        n178 = Select(t=w317, s=w318, f=w316) -> (s? t:f=w315:dbl)
        n179 = Multiply(x=w305, y=1.3) -> (x*y=w306:dbl)
        n180 = Absolute Value(x=w306) -> (abs(x)=w312:dbl)
        n181 = Absolute Value(x=w314) -> (abs(x)=w313:dbl)
        n182 = Greater Or Equal?(x=w313, y=w312) -> (x >= y?=w311:bool)
        n183 = call-poly <vilib>:"WPI_RobotDriveArcadeDrive.vi"("Y axis value"=w315, "X axis value"=0.0 ("Y axis value"), "RobotDriveDevRef"=w324) -> ()  [unwired: 6 in, 3 out]
        n184 = Select(t=TargetState."Stop" ("TargetState"), s=w311, f=TargetState."MoveToTarget" ("TargetState")) -> (s? t:f=w322:T1)
      }
      frame "ReAlign" {
        # "Y-direction"
        # "turn speed"
        # "X direction: left/right"
        # "Is target centered?"
        n185 = Index Array(array=w337, index #1=2 ("index"), index #2=1 ("index")) -> (element #1=w342:dbl, element #2=w343:dbl)
        n186 = Subtract(x=w342, y=w343) -> (x-y=w341:dbl)
        n187 = Add(x=w342, y=w343) -> (x+y=w344:dbl)
        n188 = In Range and Coerce(upper limit=w344, x=w336, lower limit=w341) -> (In Range?=w338:bool)  [unwired: 1 out]
        n189 = case shown="True" w338 {
          selector: w338 -> [w353 w357]
          tunnel: [w353 w357] -> w326
          tunnel: [w351 0.0] -> w333
          tunnel: w336 -> [w350 _]
          tunnel: w344 -> [w349 _]
          tunnel: w335 -> [w347 _]
          tunnel: [0.0 w354] -> w329
          frame False {
            # "centered"
            # "pos speed\nis left"
            # "not centered; too far right?"
            n190 = Greater Or Equal?(x=w350, y=w349) -> (x >= y?=w352:bool)
            n191 = Negate(x=w347) -> (-x=w348:dbl)
            n192 = Select(t=w347, s=w352, f=w348) -> (s? t:f=w351:dbl)
          }
          frame True {
            # "Count number of alignments"
            n193 = local read "aligncount"() -> (w355:dbl)
            n194 = Increment(x=w355) -> (x+1=w354:dbl)
            "aligncount" <- w354
          }
        }
        n195 = Greater Or Equal?(x=w329, y=2.0) -> (x >= y?=w327:bool)
        n196 = call-poly <vilib>:"WPI_RobotDriveArcadeDrive.vi"("Y axis value"=0.0, "X axis value"=w333, "RobotDriveDevRef"=w345) -> ()  [unwired: 6 in, 3 out]
        n197 = And(x=w327, y=w326) -> (x .and. y?=w325:bool)
        n198 = Select(t=TargetState."Stop" ("TargetState"), s=w325, f=TargetState."ReAlign" ("TargetState")) -> (s? t:f=w331:T1)
      }
      frame "Stop" {
        w360 = 0.0 ("X axis value")
        n199 = call-poly <vilib>:"WPI_RobotDriveArcadeDrive.vi"("Y axis value"=w360, "X axis value"=w360, "RobotDriveDevRef"=w361) -> ()  [unwired: 6 in, 3 out]
        n200 = global write "Robot Global Data.vi" "HiShoot"(TRUE) -> ()
      }
      frame "Shoot" {
        n201 = global read "Robot Global Data.vi" "HiShoot"() -> (w363:bool)
        n202 = Select(t=TargetState."Shoot" ("TargetState"), s=w363, f=TargetState."Reset" ("TargetState")) -> (s? t:f=w362:T1)
      }
      frame "Reset" {
        w366 = FALSE ("ActiveTarget")
        n203 = global write "Robot Global Data.vi" "ActivateAutoTarget"(w366) -> ()
        n204 = global write "Robot Global Data.vi" "StopAutoTarget"(w366) -> ()
      }
    }
  }
